vi "Get ListSelection.lvclass.vi"(8 "error in (no error)":errorcluster, 11 "ExcuseNotesHandler in":refnum<class "ExcuseNotesHandler.lvclass">) -> (0 "error out":errorcluster, 2 "Admin_Actor.lvlib:ListSelection.lvclass":refnum<class "ListSelection.lvclass">, 3 "ExcuseNotesHandler out":refnum<class "ExcuseNotesHandler.lvclass">)   [LabVIEW 2015, in "ExcuseNotesHandler.lvclass"]
uses:
  ExcuseNotesHandler.lvclass
  Models/ListSelection/ListSelection.lvclass
  ExcuseNotesHandler.lvclass/ExcuseNotesHandler.ctl
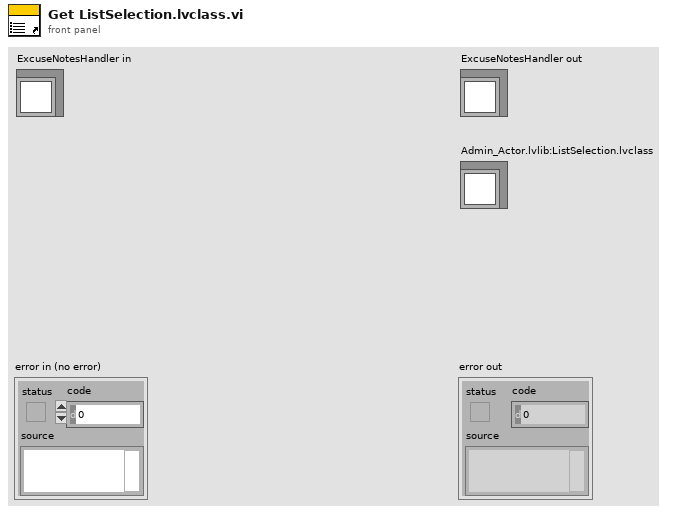
[diagram p1: front panel]
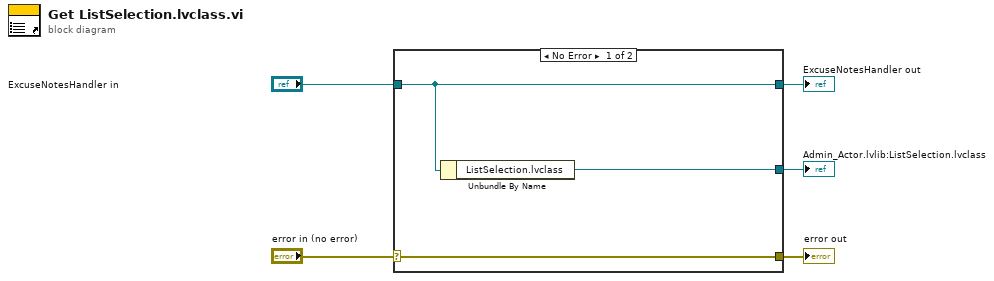
[diagram p0: block diagram]
diagram:
  n1 = case shown="No Error" "error in (no error)" {
    selector: "error in (no error)" -> [w8 w9]
    tunnel: [w8 w9] -> w4
    tunnel: [w7 w10] -> w2
    tunnel: "ExcuseNotesHandler in" -> [w7 w10]
    tunnel: [w6 _] -> w1
    frame No Error {
      n2 = Unbundle By Name(w7) -> ("ListSelection.lvclass"=w6:refnum<class "ListSelection.lvclass">)
    }
    frame Error {
    }
  }
  "error out" <- w4
  "ExcuseNotesHandler out" <- w2
  "Admin_Actor.lvlib:ListSelection.lvclass" <- w1
